vi "ziModGetTriggerData.vi"(8 "Error In":errorcluster, 10 "ModResults":T3, 11 "ModHandle In":T6 {"ModHandle" format="0x%08x"; "Conn" format="0x%08x"}) -> (0 "Error Out":errorcluster, 3 "ModHandle Out":T6 {"ModHandle" format="0x%08x"; "Conn" format="0x%08x"})   [LabVIEW 2018, in "Zurich Instruments LabOne.lvlib"]
doc: "Use this vi to get Trigger Data from a ModResult returned from ziModGetNextNode.vi. It returns an array of Trigger Data."
uses:
  Zurich Instruments LabOne.lvlib
  <instrlib>/Zurich Instruments LabOne/Private/ziLV64.framework
  Data/ziTypeTriggerSample.ctl
  Data/ziTypeTriggerSampleGrid.ctl
  ziTypeModHandle.ctl
  ziTypeModResults.ctl
  Data/ziTypePollType.ctl
  ziTypeModGenericHeader.ctl
panel:
  out "ModTriggerData":T1[](array[typedef])
  out "ModCntDataGrid":T2[](array[typedef])
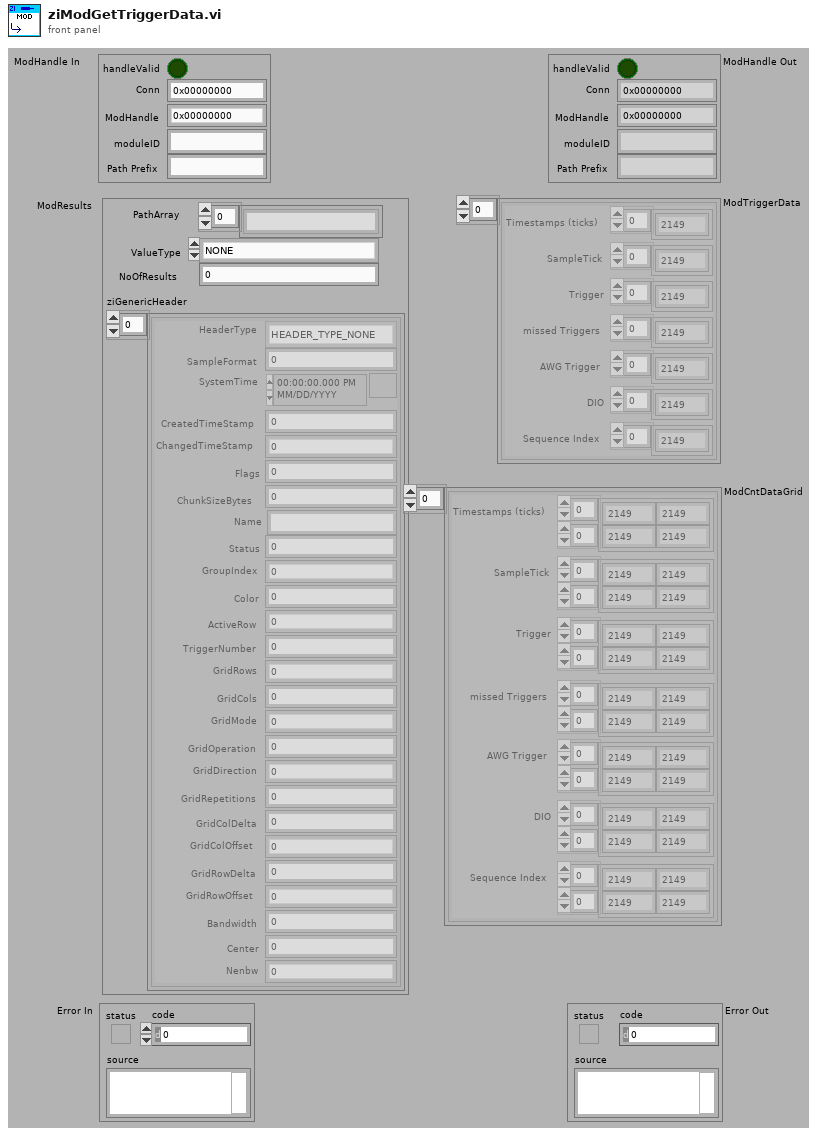
[diagram p1: front panel]
types:
  T1 = typedef "Zurich Instruments LabOne.lvlib/ziTypeTriggerSample.ctl" = cluster{"timeStamp":u64[], "sampleTick":u64[], "trigger":u32[], "missedTriggers":u32[], "awgTrigger":u32[], "dio":u32[], "sequenceIndex":u32[]}
  T2 = typedef "Zurich Instruments LabOne.lvlib/ziTypeTriggerSampleGrid.ctl" = cluster{"timeStamp":u64[][], "sampleTick":u64[][], "trigger":u32[][], "missedTriggers":u32[][], "awgTrigger":u32[][], "dio":u32[][], "sequenceIndex":u32[][]}
  T3 = typedef "Zurich Instruments LabOne.lvlib/ziTypeModResults.ctl" = cluster{"PathArray":string[], "ValueType":T4, "NoOfResults":u64, "ziGenericHeader":T5[]}
  T4 = typedef "Zurich Instruments LabOne.lvlib/ziTypePollType.ctl" = enum16{"NONE", "DOUBLE_DATA", "INTEGER_DATA", "DEMOD_SAMPLE", "SCOPE_WAVE_HF2", "AUXIN_SAMPLE", "DIO_SAMPLE", "BYTE_ARRAY", "PWA_WAVE", "9", "10", "11", "12", "13", "14", "15", "TREE_CHANGE_DEPRI", "17", "ERROR", "19", "20", "21", "22", "23", "24", "25", "26", "27", "28", "29", "30", "31", "DOUBLE_DATA_TS", "INTEGER_DATA_TS", "34", "SCOPE_WAVE", "SCOPE_WAVE_EX", "37", "BYTE_ARRAY_TS", "39", "40", "41", "42", "43", "44", "45", "CNT_DATA", "47", "TREE_CHANGE", "49", "50", "51", "52", "53", "54", "55", "56", "57", "58", "59", "60", "61", "62", "63", "SWEEPER_DATA", "SPECTRUM_DATA", "ADVISOR_DATA", "VECTOR_DATA", "IMP_DATA"}
  T5 = typedef "Zurich Instruments LabOne.lvlib/ziTypeModGenericHeader.ctl" = cluster{"HeaderType":enum8{"HEADER_TYPE_NONE", "HEADER_TYPE_SWTRIGGER", "HEADER_TYPE_SWEEPER"}, "SampleFormat":u8, "SystemTime":timestamp, "CreatedTimeStamp":u64, "ChangedTimeStamp":u64, "Flags":u32, "ChunkSizeBytes":u64, "Name":string, "Status":u32, "GroupIndex":u32, "Color":u32, "ActiveRow":u32, "TriggerNumber":u64, "GridRows":u32, "GridCols":u32, "GridMode":u32, "GridOperation":u32, "GridDirection":u32, "GridRepetitions":u32, "GridColDelta":dbl, "GridColOffset":dbl, "GridRowDelta":dbl, "GridRowOffset":dbl, "Bandwidth":dbl, "Center":dbl, "Nenbw":dbl}
  T6 = typedef "Zurich Instruments LabOne.lvlib/ziTypeModHandle.ctl" = cluster{"handleValid":bool, "Conn":u64, "ModHandle":u64, "moduleID":string, "Path Prefix":string}
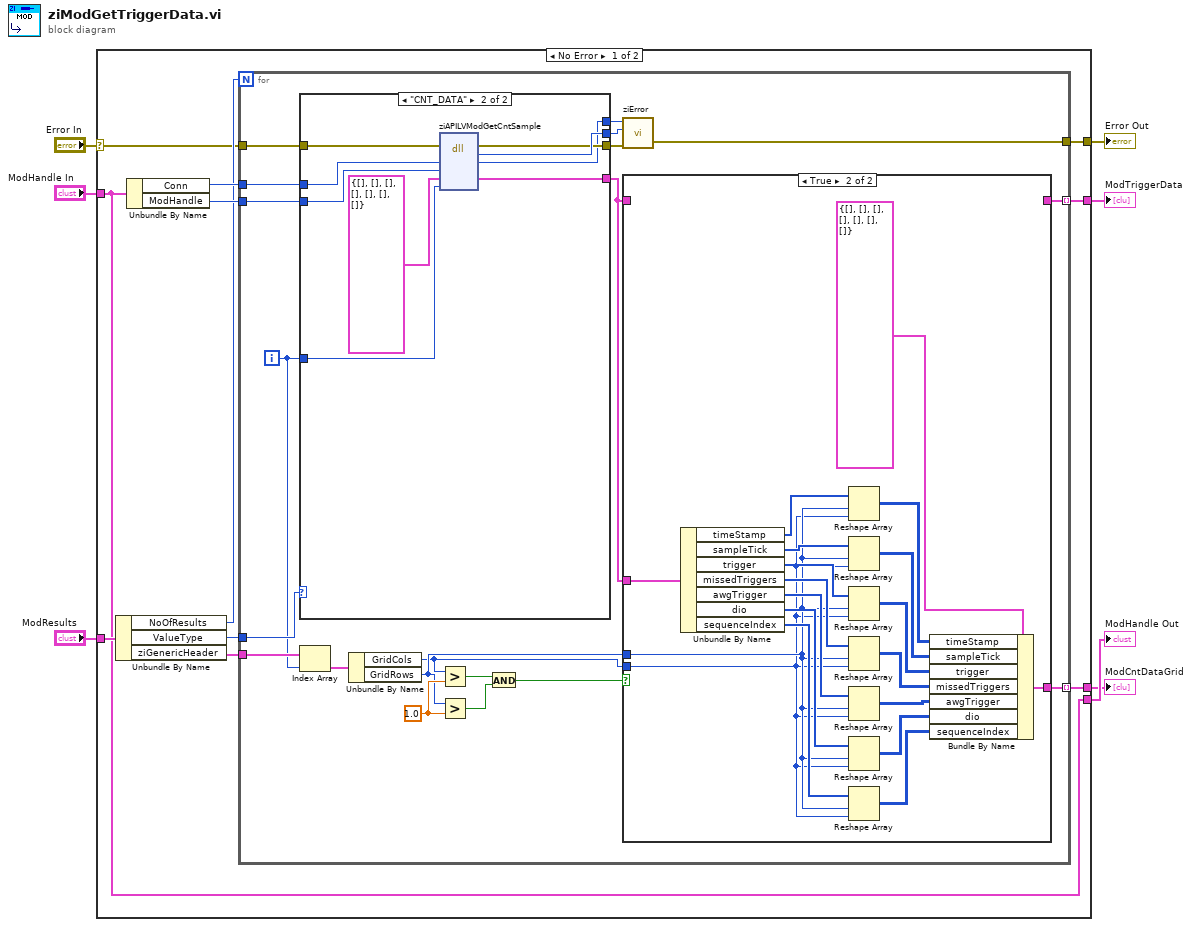
[diagram p0: block diagram]
diagram:
  n1 = case shown="No Error" "Error In" {
    selector: "Error In" -> [w13 w70]
    tunnel: [w14 w70] -> w3
    tunnel: [w12 w71] -> w6
    tunnel: "ModHandle In" -> [w12 w71]
    tunnel: "ModResults" -> [w16 _]
    tunnel: [w10 _] -> w2
    tunnel: [w8 _] -> w1
    frame No Error {
      n2 = Unbundle By Name(w16) -> ("NoOfResults"=w15:u64, "ValueType"=w11:T4, "ziGenericHeader"=w9:T5[])
      n3 = Unbundle By Name(w12) -> ("Conn"=w18:u64, "ModHandle"=w17:u64)
      n4 = for {
        N: w15 -> [_]
        tunnel: w18 -> [w38]
        tunnel: w17 -> [w37]
        tunnel: [w36] -> w14
        tunnel: w13 -> [w33]
        tunnel: w11 -> [w32]
        tunnel: [w24] -> w10 mode=indexing
        tunnel: w9 -> [w21]
        tunnel: [w22] -> w8 mode=indexing
        i -> [w20]
        w28 = 1.0 ("y")
        n5 = case shown="\"CNT_DATA\"" w32 {
          tunnel: w38 -> [w59 w69]
          tunnel: w37 -> [_ w68]
          tunnel: w20 -> [_ w67]
          tunnel: [_ w66] -> w35
          tunnel: [w60 w65] -> w34
          tunnel: w33 -> [w60 w64]
          tunnel: [_ w63] -> w23
          tunnel: [w59 w62] -> w31
          frame "NONE", Default {
          }
          frame "CNT_DATA" {
            n6 = dll-call lib="Applications/National Instruments/LabVIEW 2019 64-bit/instr.lib/Zurich Instruments LabOne/Private/ziLV*.*" fn="ziAPILVModGetCntSample"(error in=w64, "Conn"=w69, "ModHandle"=w68, "DEMODData"=T1 {"timeStamp"=[], "sampleTick"=[], "trigger"=[], "missedTriggers"=[], "awgTrigger"=[], "dio"=[], "sequenceIndex"=[]} ("Trigger Sample"), "chunk_idx"=w67) -> (error out=w65:errorcluster, "return type"=w66:u32, "Conn"=w62:u64, "DEMODData"=w63:T1)  [unwired: 4 in, 1 out]
          }
        }
        n7 = Index Array(array=w21, index=w20) -> (element=w19:T5)
        n8 = Unbundle By Name(w19) -> ("GridCols"=w26:u32, "GridRows"=w27:u32)
        n9 = Greater?(x=w26, y=w28) -> (0:w30:bool)
        n10 = Greater?(x=w27, y=w28) -> (0:w29:bool)
        n11 = And(x=w30, y=w29) -> (x .and. y?=w25:bool)
        n12 = call "ziError.vi"("Conn"=w31, "ziErrorCode"=w35, "Error In"=w34) -> ("Error Out"=w36:errorcluster)  [unwired: 2 in, 1 out]
        n13 = case shown="True" w25 {
          tunnel: w23 -> [_ w58]
          tunnel: w23 -> [w39 _]
          tunnel: [w39 _] -> w24
          tunnel: w27 -> [_ w43]
          tunnel: w26 -> [_ w42]
          tunnel: [_ w57] -> w22
          frame False {
          }
          frame True {
            n14 = Unbundle By Name(w58) -> ("timeStamp"=w44:u64[], "sampleTick"=w45:u64[], "trigger"=w46:u32[], "missedTriggers"=w47:u32[], "awgTrigger"=w48:u32[], "dio"=w54:u32[], "sequenceIndex"=w55:u32[])
            n15 = Reshape Array(w44, w43, w42) -> (w49:u64[][])
            n16 = Reshape Array(w45, w43, w42) -> (w50:u64[][])
            n17 = Reshape Array(w46, w43, w42) -> (w51:u32[][])
            n18 = Reshape Array(w47, w43, w42) -> (w41:u32[][])
            n19 = Reshape Array(w48, w43, w42) -> (w40:u32[][])
            n20 = Reshape Array(w54, w43, w42) -> (w52:u32[][])
            n21 = Reshape Array(w55, w43, w42) -> (w53:u32[][])
            n22 = Bundle By Name(cluster=T2 {"timeStamp"=[], "sampleTick"=[], "trigger"=[], "missedTriggers"=[], "awgTrigger"=[], "dio"=[], "sequenceIndex"=[]} ("Trigger Sample"), "timeStamp"=w49, "sampleTick"=w50, "trigger"=w51, "missedTriggers"=w41, "awgTrigger"=w40, "dio"=w52, "sequenceIndex"=w53) -> (w57:T2)
          }
        }
      }
    }
    frame Error {
    }
  }
  "Error Out" <- w3
  "ModHandle Out" <- w6
  "ModCntDataGrid" <- w1
  "ModTriggerData" <- w2
